vi "Persistent.vi"(7 "Field monitor ref":refnum<vi>, 8 "error in (no error)":errorcluster, 10 "Go to persistent mode?":bool, 11 "Power Supply in":refnum<class "Power Supply.lvclass">) -> (0 "error out":errorcluster, 3 "Power Supply out":refnum<class "Power Supply.lvclass">)   [LabVIEW 2023, in "Power Supply.lvclass"]
doc: "Persistent mode closes the switch and turns off the power supply. The superconducting electromagnet will then remain energized indefinitely.\n\nTo leave persistent mode, you must first ramp up the power supply to match the energized magnet, then open the switch. \n\nA current mismatch is dangerous! The magnet will forbid opening the switch unless the power supply matches the energized magnet."
uses:
  Power Supply.lvclass
  Global/Relative Sound Files.vi
panel:
  out "Power supply output \"field\"":dbl[unit]
  out "SHon?":bool caption="Switch Heater"
  out "persis?":bool caption="Persistent"
  out "title":string
  out "Field":dbl[unit]
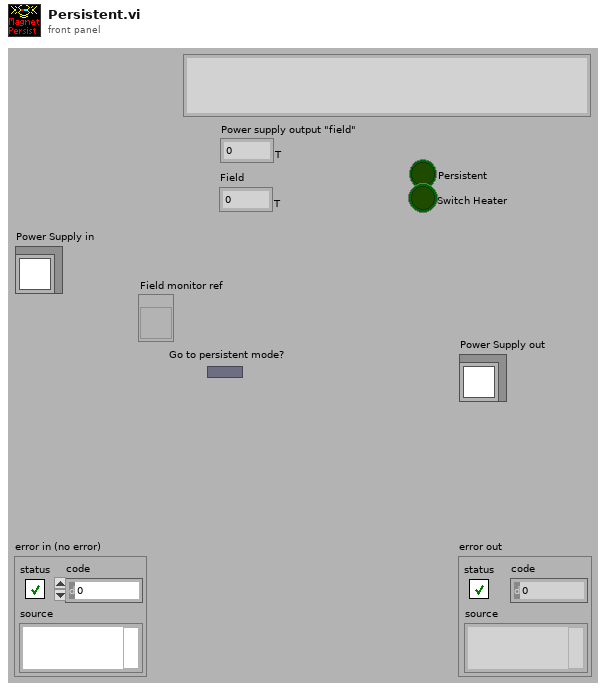
[diagram p1: front panel]
types:
  T1 = typedef "Power Supply.lvclass/Switch Heater Status.ctl" = enum16{"Off (at zero)", "On", "Off (at field)", "Other"}
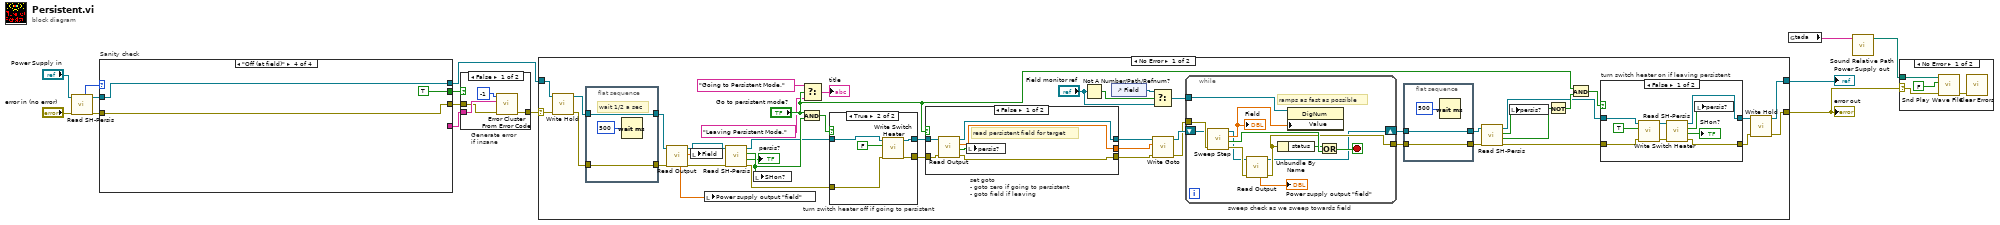
[diagram p0: block diagram]
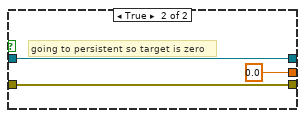
[diagram p3: hidden frame]
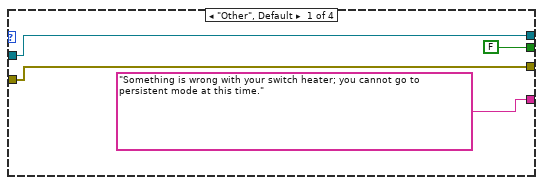
[diagram p7: hidden frame]
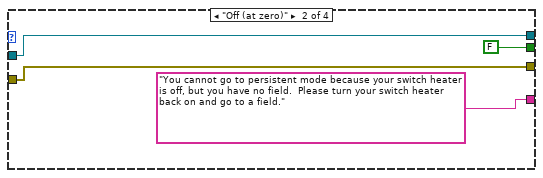
[diagram p8: hidden frame]
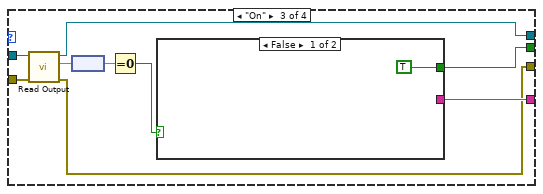
[diagram p9: hidden frame]
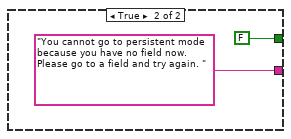
[diagram p10: hidden frame]
diagram:
  n1 = call-dynamic "Read SH-Persis.vi"("error in (no error)"="error in (no error)", "Power Supply in"="Power Supply in") -> ("error out"=w6:errorcluster, "Power Supply out"=w8:refnum<class "Power Supply.lvclass">, "SHstatus"=w11:T1)  [unwired: 4 in, 3 out]
  n2 = case "Sanity check" shown="\"Off (at field)\"" w11 {
    tunnel: [FALSE FALSE w31 TRUE] -> w10
    tunnel: ["Something is wrong with your switch heater; you cannot go to persistent mode at this time." "You cannot go to persistent mode because your switch heater is off, but you have no field.  Please turn your switch heater back on and go to a field." w28 _] -> w9
    tunnel: w8 -> [w16 w20 w27 w36]
    tunnel: [w16 w20 w26 w36] -> w12
    tunnel: [w15 w19 w25 w35] -> w7
    tunnel: w6 -> [w15 w19 w24 w35]
    frame "Other", Default {
    }
    frame "Off (at zero)" {
    }
    frame "On" {
      n3 = call-dynamic "Read Output.vi"("error in (no error)"=w24, "Power Supply in"=w27) -> ("error out"=w25:errorcluster, "Field"=w30:dbl[unit], "Power Supply out"=w26:refnum<class "Power Supply.lvclass">)  [unwired: 5 in, 2 out]
      n4 = node(w30) -> (w23:dbl)
      n5 = Equal To 0?(x=w23) -> (x = 0?=w29:bool)
      n6 = case shown="False" w29 {
        tunnel: [TRUE FALSE] -> w31
        tunnel: [_ "You cannot go to persistent mode because you have no field now.  Please go to a field and try again. "] -> w28
        frame False {
        }
        frame True {
        }
      }
    }
    frame "Off (at field)" {
    }
  }
  n7 = case "Generate error\nif insane" shown="False" w10 {
    tunnel: w9 -> [w40 _]
    tunnel: [w39 w42] -> w4
    tunnel: w7 -> [w38 w42]
    frame False {
      n8 = call <vilib>:"Error Cluster From Error Code.vi"("error in (no error)"=w38, "error message (\"\")"=w40, "error code (0)"=-1) -> ("error out"=w39:errorcluster)  [unwired: 6 in]
    }
    frame True {
    }
  }
  n9 = case shown="No Error" w4 {
    selector: w4 -> [w48 w133]
    tunnel: [w85 w132] -> w13
    tunnel: [w84 w133] -> w3
    tunnel: w12 -> [w53 w132]
    frame No Error {
      n10 = call-dynamic "Write Hold.vi"("error in (no error)"=w48, "Power Supply in"=w53) -> ("error out"=w49:errorcluster, "Power Supply out"=w52:refnum<class "Power Supply.lvclass">)  [unwired: 8 in]
      n11 = flat-sequence {
        tunnel: w52 -> [w89]
        tunnel: [w89] -> w51
        tunnel: [w88] -> w50
        tunnel: w49 -> [w88]
        frame #0 {
          # "wait 1/2 a sec"
          n12 = Wait (ms)(milliseconds to wait=500) -> ()  [unwired: 1 out]
        }
      }
      n13 = call-dynamic "Read Output.vi"("error in (no error)"=w50, "Power Supply in"=w51) -> ("error out"=w60:errorcluster, "Field"=w54:dbl[unit], "Power Supply out"=w61:refnum<class "Power Supply.lvclass">, "Power supply \"field\""=w43:dbl[unit])  [unwired: 5 in, 1 out]
      n14 = local write "Field"(w54) -> ()
      n15 = local write "Power supply output \"field\""(w43) -> ()
      n16 = call-dynamic "Read SH-Persis.vi"("error in (no error)"=w60, "Power Supply in"=w61) -> ("error out"=w58:errorcluster, "SHon?"=w63:bool, "pers?"=→"persis?":bool, "Power Supply out"=w59:refnum<class "Power Supply.lvclass">)  [unwired: 4 in, 2 out]
      n17 = local write "SHon?"(w63) -> ()
      n18 = And(x="Go to persistent mode?", y=w63) -> (x .and. y?=w64:bool)
      n19 = Select(t="Going to Persistent Mode.", s="Go to persistent mode?", f="Leaving Persistent Mode.") -> (s? t:f=→"title":string)
      n20 = case "turn switch heater off if going to persistent" shown="True" w64 {
        tunnel: [w91 w94] -> w67
        tunnel: w59 -> [w91 w95]
        tunnel: w58 -> [w90 w93]
        tunnel: [w90 w92] -> w66
        frame False {
        }
        frame True {
          n21 = call-dynamic "Write Switch Heater.vi"("error in (no error)"=w93, "Turn SH On?"=FALSE, "Power Supply in"=w95) -> ("error out"=w92:errorcluster, "Power Supply out"=w94:refnum<class "Power Supply.lvclass">)  [unwired: 7 in]
        }
      }
      n22 = case "set goto\n- goto zero if going to persistent\n- goto field if leaving" shown="False" "Go to persistent mode?" {
        tunnel: [w101 dbl[unit] 0.0 ("Field")] -> w69
        tunnel: [w100 w104] -> w68
        tunnel: w67 -> [w99 w104]
        tunnel: w66 -> [w98 w103]
        tunnel: [w97 w103] -> w65
        frame False {
          # "read persistent field for target"
          n23 = call-dynamic "Read Output.vi"("error in (no error)"=w98, "Power Supply in"=w99) -> ("error out"=w97:errorcluster, "persistent?"=w102:bool, "Field"=w101:dbl[unit], "Power Supply out"=w100:refnum<class "Power Supply.lvclass">)  [unwired: 5 in, 1 out]
          n24 = local write "persis?"(w102) -> ()
        }
        frame True {
          # "going to persistent so target is zero"
        }
      }
      n25 = Not A Number/Path/Refnum?(number/path/refnum="Field monitor ref") -> (NaN/Path/Refnum?=w47:bool)
      n26 = control-ref of="Field"() -> (w46:refnum<vi>)
      n27 = Select(t=w46, s=w47, f="Field monitor ref") -> (s? t:f=w44:refnum<vi>)
      n28 = call-dynamic "Write Goto.vi"("error in (no error)"=w65, "Target"=w69, "Power Supply in"=w68) -> ("error out"=w70:errorcluster, "Power Supply out"=w71:refnum<class "Power Supply.lvclass">)  [unwired: 7 in]
      n29 = while "sweep check as we sweep towards field" {
        shift-right: [w107] -> w73
        shift-left: w71 -> [w111]
        tunnel: [w110] -> w72
        tunnel: w70 -> [w116]
        tunnel: w44 -> [w115]
        stop <- w113 stop-if-true
        # "ramps as fast as possible"
        n30 = call-dynamic "Sweep Step.vi"("error in (no error)"=w116, "Power Supply in"=w111) -> ("error out"=w109:errorcluster, "Done?"=w117:bool, "field"=w114:dbl[unit], "Power Supply out"=w108:refnum<class "Power Supply.lvclass">)  [unwired: 5 in, 1 out]
        "Field" <- w114
        n31 = call-dynamic "Read Output.vi"("error in (no error)"=w109, "Power Supply in"=w108) -> ("error out"=w110:errorcluster, "Power Supply out"=w107:refnum<class "Power Supply.lvclass">, "Power supply \"field\""=→"Power supply output \"field\"":dbl[unit])  [unwired: 5 in, 2 out]
        n32 = Unbundle By Name(w110) -> ("status"=w112:bool)
        n33 = property on="Property Node" class="DigNum"(reference=w115, "Value"=w114) -> ()  [unwired: 1 in, 2 out]
        n34 = Or(x=w112, y=w117) -> (x .or. y?=w113:bool)
      }
      n35 = flat-sequence {
        tunnel: w73 -> [w119]
        tunnel: [w119] -> w77
        tunnel: w72 -> [w118]
        tunnel: [w118] -> w76
        frame #0 {
          n36 = Wait (ms)(milliseconds to wait=500) -> ()  [unwired: 1 out]
        }
      }
      n37 = call-dynamic "Read SH-Persis.vi"("error in (no error)"=w76, "Power Supply in"=w77) -> ("error out"=w75:errorcluster, "SHon?"=w79:bool, "pers?"=w78:bool, "Power Supply out"=w74:refnum<class "Power Supply.lvclass">)  [unwired: 4 in, 2 out]
      n38 = local write "persis?"(w78) -> ()
      n39 = Not(x=w79) -> (.not. x?=w80:bool)
      n40 = And(x="Go to persistent mode?", y=w80) -> (x .and. y?=w81:bool)
      n41 = case "turn switch heater on if leaving persistent" shown="False" w81 {
        tunnel: [w125 w130] -> w82
        tunnel: w75 -> [w128 w130]
        tunnel: w74 -> [w129 w131]
        tunnel: [w121 w131] -> w83
        frame False {
          n42 = call-dynamic "Write Switch Heater.vi"("error in (no error)"=w128, "Turn SH On?"=TRUE, "Power Supply in"=w129) -> ("error out"=w126:errorcluster, "Power Supply out"=w122:refnum<class "Power Supply.lvclass">)  [unwired: 7 in]
          n43 = call-dynamic "Read SH-Persis.vi"("error in (no error)"=w126, "Power Supply in"=w122) -> ("error out"=w125:errorcluster, "SHon?"=→"SHon?":bool, "pers?"=w123:bool, "Power Supply out"=w121:refnum<class "Power Supply.lvclass">)  [unwired: 4 in, 2 out]
          n44 = local write "persis?"(w123) -> ()
        }
        frame True {
        }
      }
      n45 = call-dynamic "Write Hold.vi"("error in (no error)"=w82, "Power Supply in"=w83) -> ("error out"=w84:errorcluster, "Power Supply out"=w85:refnum<class "Power Supply.lvclass">)  [unwired: 8 in]
    }
    frame Error {
    }
  }
  "Power Supply out" <- w13
  "error out" <- w3
  n46 = global read "Relative Sound Files.vi" "tada"() -> (w2:string)
  n47 = call "Sound Relative Path.vi"("Sound"=w2) -> ("Relative Path"=w1:path)  [unwired: 10 in]
  n48 = case shown="No Error" w3 {
    selector: w3 -> [w134 _]
    tunnel: w1 -> [w137 _]
    frame No Error {
      n49 = call <vilib>:"Snd Play Wave File.vi"("error in (no error)"=w134, "wait until finish (T)"=FALSE, "wave file path"=w137) -> ("error out"=w135:errorcluster)  [unwired: 8 out]
      n50 = call <vilib>:"Clear Errors.vi"("error in (no error)"=w135) -> ()  [unwired: 5 in, 2 out]
    }
    frame Error {
    }
  }
